vi "ExperimentSettings.vi"(4 "small?":bool, 5 "Experiment Settings id":u16, 6 "Enable":bool, 7 "Default Experiment Name":string caption="Please Enter Tags:", 8 "error in (no error)":errorcluster, 9 "current time":timestamp, 10 "default Experiment Description":string caption="Please Enter Experiment Description:", 11 "Default Group ID":u16(ring) items=["CCLDAS"=1, "LASP"=2, "CU"=3, "NLSI"=4, "LDEX"=5, "Heidelberg"=6]) -> (0 "error out":errorcluster, 3 "output cluster":T1)   [LabVIEW 2013]
uses:
  Public API/ExperimentSetting.ctl
  <vilib>/addons/database/NI_Database_API.lvlib
panel:
  in  "ExperimentSetting":T1
  # "Experiment Settings"
  # "Experiment Settings"
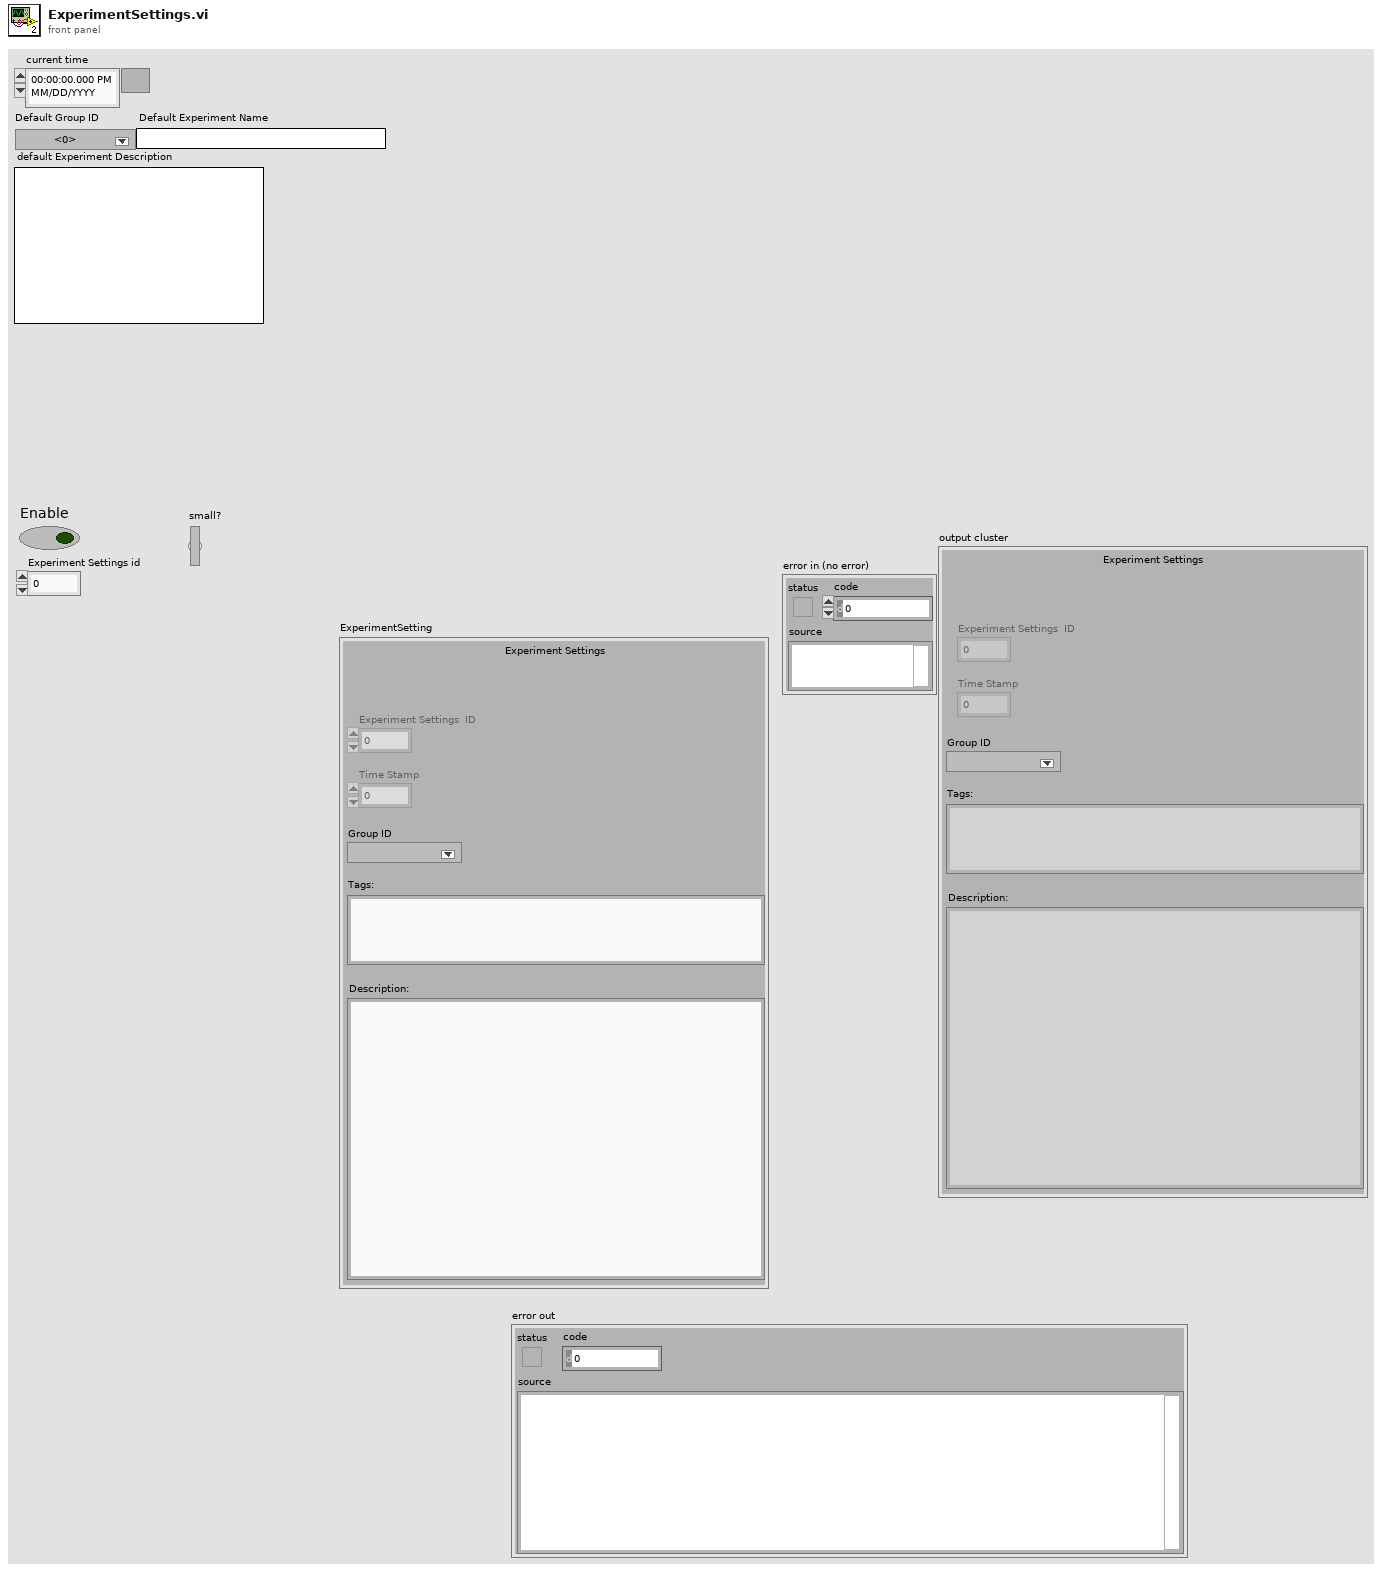
[diagram p1: front panel]
types:
  T1 = typedef "ExperimentSetting.ctl" = cluster{"Experiment Settings  ID":i64, "Time Stamp":i64, "Group ID":i32, "Tags:":string, "Description:":string}
  T2 = cluster{"Please Enter Tags:":string, "Please Enter Experiment Description:":string, "Default Group ID":i32}
  T3 = typedef "NI_Database_API.lvlib/Conn ObjectReference.ctl" = refnum<k1>
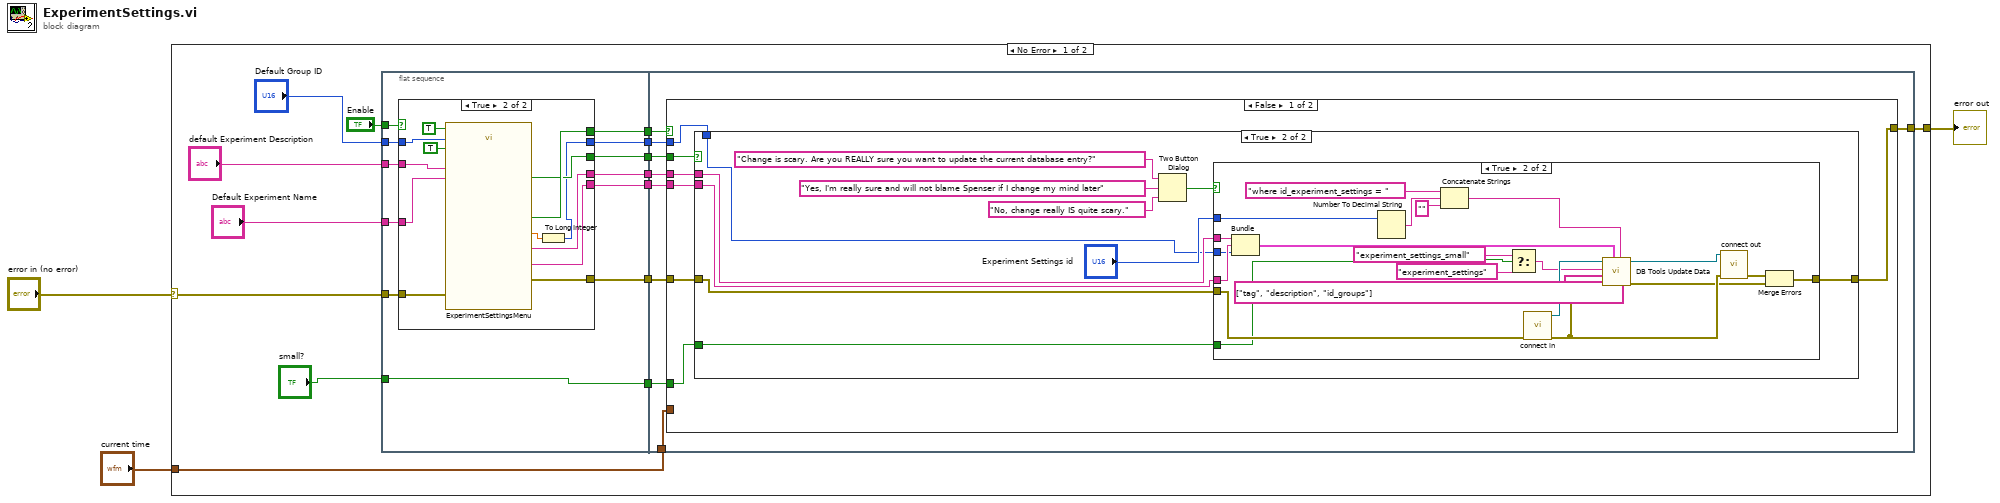
[diagram p0: block diagram]
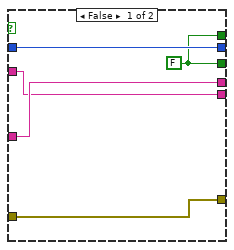
[diagram p2: hidden frame]
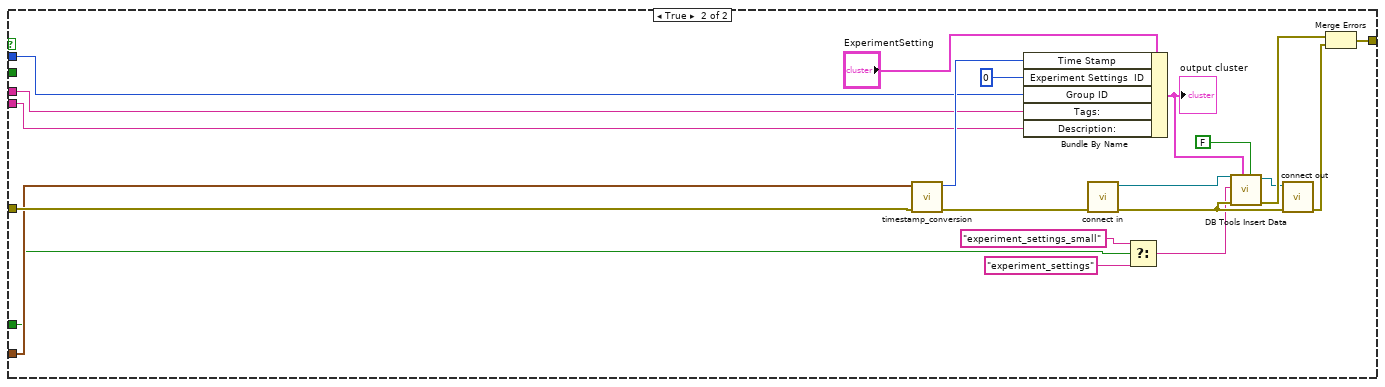
[diagram p5: hidden frame]
diagram:
  n1 = case shown="No Error" "error in (no error)" {
    selector: "error in (no error)" -> [w18 w120]
    tunnel: [w13 w120] -> w2
    tunnel: "current time" -> [w8 _]
    frame No Error {
      n2 = flat-sequence {
        tunnel: w18 -> [w30]
        tunnel: [w29] -> w17
        tunnel: [w28] -> w16
        tunnel: [w27] -> w15
        tunnel: [w26] -> w14
        tunnel: "Default Group ID" -> [w22]
        tunnel: "default Experiment Description" -> [w25]
        tunnel: "Default Experiment Name" -> [w24]
        tunnel: [w20] -> w9
        tunnel: "Enable" -> [w23]
        tunnel: [w19] -> w6
        tunnel: [w21] -> w5
        tunnel: "small?" -> [w21]
        tunnel: w17 -> [w57]
        tunnel: w16 -> [w56]
        tunnel: w15 -> [w55]
        tunnel: w14 -> [w54]
        tunnel: w9 -> [w52]
        tunnel: w8 -> [w51]
        tunnel: w6 -> [w50]
        tunnel: w5 -> [w49]
        tunnel: [w53] -> w13
        frame #0 {
          n3 = case shown="True" w23 {
            tunnel: w30 -> [w32 w48]
            tunnel: [w32 w47] -> w29
            tunnel: [w33 w46] -> w28
            tunnel: [w34 w45] -> w27
            tunnel: [w35 w37] -> w26
            tunnel: w22 -> [w35 w44]
            tunnel: w25 -> [w33 w43]
            tunnel: w24 -> [w34 w42]
            tunnel: [w31 w40] -> w20
            tunnel: [w31 w39] -> w19
            frame False {
              w31 = FALSE ("Cancel 2")
            }
            frame True {
              n4 = call "ExperimentSettingsMenu.vi"("Enable"=TRUE, "Default Group ID"=w44, "sub vi?"=TRUE, "error in (no error)"=w48, "Default Experiment Name"=w42, "default Experiment Description"=w43) -> ("Update"=w39:bool, "Please Enter Experiment Description:"=w46:string, "Please Enter Tags:"=w45:string, "Please Enter Group ID"=w38:dbl, "New"=w40:bool, "error out"=w47:errorcluster)  [unwired: 7 in, 1 out]
              n5 = To Long Integer(number=w38) -> (32bit integer=w37:i32)
            }
          }
        }
        frame #1 {
          n6 = case shown="False" w52 {
            tunnel: w57 -> [w64 w108]
            tunnel: w56 -> [w61 w107]
            tunnel: w55 -> [w62 w106]
            tunnel: w54 -> [w59 w105]
            tunnel: [w63 w104] -> w53
            tunnel: w51 -> [_ w103]
            tunnel: w50 -> [w60 _]
            tunnel: w49 -> [w58 w100]
            frame False {
              n7 = case shown="True" w60 {
                tunnel: w64 -> [w65 w76]
                tunnel: [w65 w75] -> w63
                tunnel: w62 -> [_ w74]
                tunnel: w61 -> [_ w73]
                tunnel: w59 -> [_ w67]
                tunnel: w58 -> [_ w66]
                frame False {
                }
                frame True {
                  n8 = Two Button Dialog(message="Change is scary. Are you REALLY sure you want to update the current database entry?", 1:"No, change really IS quite scary." ("F button name (\"Cancel\")"), 2:"Yes, I'm really sure and will not blame Spenser if I change my mind later" ("T button name (\"OK\")")) -> (T button?=w71:bool)
                  n9 = case shown="True" w71 {
                    tunnel: w76 -> [w77 w84]
                    tunnel: [w77 w87] -> w75
                    tunnel: w74 -> [_ w93]
                    tunnel: w73 -> [_ w92]
                    tunnel: "Experiment Settings id" -> [_ w95]
                    tunnel: w67 -> [_ w82]
                    tunnel: w66 -> [_ w80]
                    frame False {
                    }
                    frame True {
                      n10 = Bundle("Please Enter Tags:"=w93, "Please Enter Experiment Description:"=w92, "Default Group ID"=w82) -> (w91:T2)  [unwired: 1 in]
                      n11 = Number To Decimal String(number=w95) -> (decimal integer string=w97:string)  [unwired: 1 in]
                      n12 = Concatenate Strings("where id_experiment_settings = " ("condition"), w97, "" ("string")) -> (w94:string)
                      n13 = Select(t="experiment_settings_small" ("table"), s=w80, f="experiment_settings" ("table")) -> (s? t:f=w78:string)
                      n14 = call "connect in.vi"("error in (no error)"=w84) -> ("error out"=w90:errorcluster, "Database Connection"=w88:T3)  [unwired: 6 in, 1 out]
                      n15 = call <vilib>:"DB Tools Update Data.vi"("condition"=w94, "data"=w91, "error in (no error)"=w90, "columns"=string[] ["tag", "description", "id_groups"], "table"=w78, "connection reference"=w88) -> ("error out"=w85:errorcluster, "connection reference out"=w89:T3)  [unwired: 4 in]
                      n16 = call "connect out.vi"("error in (no error)"=w90, "connection reference"=w89) -> ("error out"=w86:errorcluster)  [unwired: 9 in]
                      n17 = Merge Errors(w86, w85) -> (w87:errorcluster)
                    }
                  }
                }
              }
            }
            frame True {
              n18 = call "timestamp_conversion.vi"("error in (no error)"=w108, "Time Stamp"=w103) -> ("error out"=w118:errorcluster, "Integer Time"=w116:i64)  [unwired: 7 in]
              n19 = Bundle By Name(cluster="ExperimentSetting", "Time Stamp"=w116, "Experiment Settings  ID"=i64 0, "Group ID"=w105, "Tags:"=w106, "Description:"=w107) -> (w119:T1)
              "output cluster" <- w119
              n20 = call "connect in.vi"("error in (no error)"=w118) -> ("error out"=w113:errorcluster, "Database Connection"=w109:T3)  [unwired: 6 in, 1 out]
              n21 = Select(t="experiment_settings_small" ("table"), s=w100, f="experiment_settings" ("table")) -> (s? t:f=w101:string)
              n22 = call <vilib>:"DB Tools Insert Data.vi"("create table? (F)"=FALSE, "data"=w119, "error in (no error)"=w113, "table"=w101, "connection reference"=w109) -> ("error out"=w112:errorcluster, "connection reference out"=w111:T3)  [unwired: 5 in]
              n23 = call "connect out.vi"("error in (no error)"=w113, "connection reference"=w111) -> ("error out"=w114:errorcluster)  [unwired: 9 in]
              n24 = Merge Errors(w112, w114) -> (w104:errorcluster)
            }
          }
        }
      }
    }
    frame Error {
    }
  }
  "error out" <- w2
